vi "triangular waveform.vi"(8 "Increasing?":bool, 9 "# of steps":dbl, 10 "max":dbl, 11 "min":dbl) -> (3 "data":dbl[](array[numeric]))   [LabVIEW 2012]
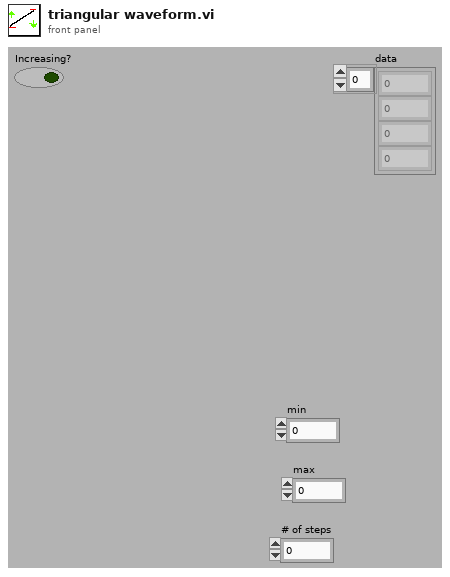
[diagram p1: front panel]
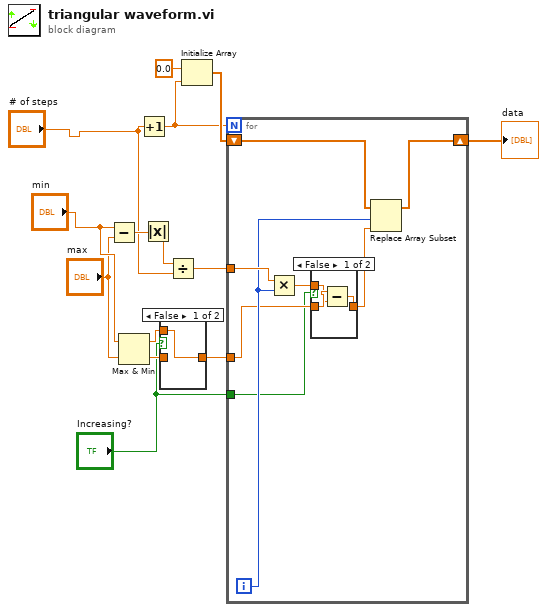
[diagram p0: block diagram]
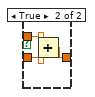
[diagram p3: hidden frame]
diagram:
  n1 = Subtract(x="min", y="max") -> (x-y=w14:dbl)
  n2 = Max & Min(x="min", y="max") -> (max(x,y)=w3:dbl, min(x,y)=w5:dbl)
  n3 = Increment(x="# of steps") -> (x+1=w6:dbl)
  n4 = Absolute Value(x=w14) -> (abs(x)=w13:dbl)
  n5 = case shown="False" "Increasing?" {
    tunnel: w5 -> [_ w16]
    tunnel: [w15 w16] -> w4
    tunnel: w3 -> [w15 _]
    frame False {
    }
    frame True {
    }
  }
  n6 = Divide(x=w13, y="# of steps") -> (x/y=w10:dbl)
  n7 = Initialize Array(0.0 ("element"), w6) -> (w8:dbl[])
  n8 = for {
    N: w6 -> [_]
    tunnel: w4 -> [w19]
    tunnel: w10 -> [w24]
    shift-right: [w21] -> w7
    shift-left: w8 -> [w22]
    tunnel: "Increasing?" -> [w17]
    i -> [w23]
    n9 = Multiply(x=w24, y=w23) -> (x*y=w18:dbl)
    n10 = case shown="False" w17 {
      tunnel: w19 -> [w27 w29]
      tunnel: [w25 w28] -> w20
      tunnel: w18 -> [w26 w30]
      frame False {
        n11 = Subtract(x=w27, y=w26) -> (x-y=w25:dbl)
      }
      frame True {
        n12 = Add(x=w30, y=w29) -> (x+y=w28:dbl)
      }
    }
    n13 = Replace Array Subset(array=w22, new element=w20, index=w23) -> (w21:dbl[])
  }
  "data" <- w7
